vi "PXI-Reset.vi"(8 "error in (no error)":errorcluster, 11 "Clear signal bank (F)":bool) -> (0 "error out":errorcluster)   [LabVIEW 2020]
doc: "Performs common PXI DAQ initialization tasks. Simplifies configuration process in higher-level measurement VIs."
uses:
  Type Defs/PXI-DO Signal Bank Action.ctl
  DAQ Engine VIs/PXI Globals.vi
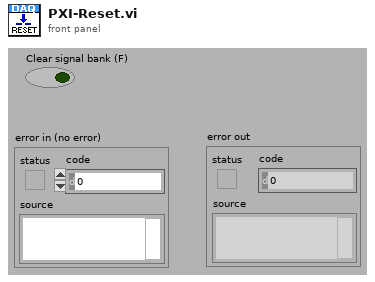
[diagram p1: front panel]
types:
  T1 = typedef "PXI-DO Signal Bank Action.ctl" = enum16{"Clear", "Write", "Read"}
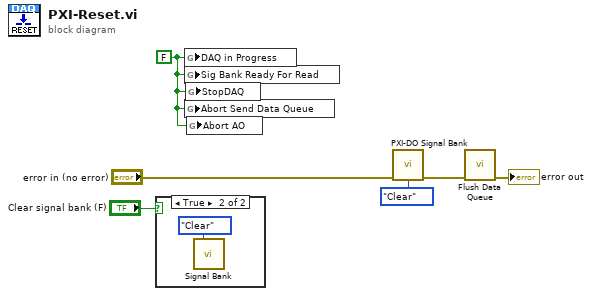
[diagram p0: block diagram]
diagram:
  w4 = FALSE ("DAQ in Progress")
  n1 = case shown="True" "Clear signal bank (F)" {
    frame False {
    }
    frame True {
      n2 = call "Signal Bank.vi"("Action"=enum16{"Add", "Replace ID", "Read ID", "Clear"}."Clear") -> ()  [unwired: 13 in, 2 out]
    }
  }
  n3 = global write "PXI Globals.vi" "DAQ in Progress"(w4) -> ()
  n4 = global write "PXI Globals.vi" "Sig Bank Ready For Read"(w4) -> ()
  n5 = global write "PXI Globals.vi" "Abort Send Data Queue"(w4) -> ()
  n6 = global write "PXI Globals.vi" "StopDAQ"(w4) -> ()
  n7 = global write "PXI Globals.vi" "Abort AO"(w4) -> ()
  n8 = call "PXI-DO Signal Bank.vi"("error in (no error)"="error in (no error)", "Action"=PXI-DO_Signal_Bank_Action."Clear") -> ("error out"=w2:errorcluster)  [unwired: 12 in, 1 out]
  n9 = call "Flush Data Queue.vi"("error in (no error)"=w2) -> ("error out"=→"error out":errorcluster)  [unwired: 10 in]
